vi "main.vi"() -> ()   [LabVIEW 2014]
uses:
  <vilib>/Utility/cursorutil.llb/Set Cursor (Icon Pict).vi
  <vilib>/vision/NI_Vision_Development_Module.lvlib
panel:
  out "DXF图":T1(plugin-control)
  out "填充效果":T1(plugin-control)
  out "文本":string
  in  "DXF文件路径":path
  out "数组":bool[][](array[boolean])
  out "未处理图像":T1(plugin-control)
  # "Usage: (1) The program written in LabVIEW 2014, you need to install NI Vision (2) First open the dxf path\n           (3) after the operation shows dxf graphics, in the \"DXF\" interface, the mouse click where you need to fill can\n                be automatically filled\nNote: DXF only supports \"segment\", \"circle\", \"arc\", rectangle or polygon needs to be decomposed into DXF, DXF is \n          saved, ellipse and elliptical arc are not supported"
  # "DXF图像填充器"
  # "使用方法：（1）本程序在LabVIEW 2014中编写，需要安装NI Vision（2）先打开dxf路径\n               （3）运行之后显示出dxf图形，在“DXF图”界面鼠标点击需要填充的地方即可实现自动填充\n注意：dxf图中仅支持“线段”、“圆”、“圆弧”，矩形或多边形需要分解爆炸成线段后保存DXF，不支持椭圆及椭圆弧"
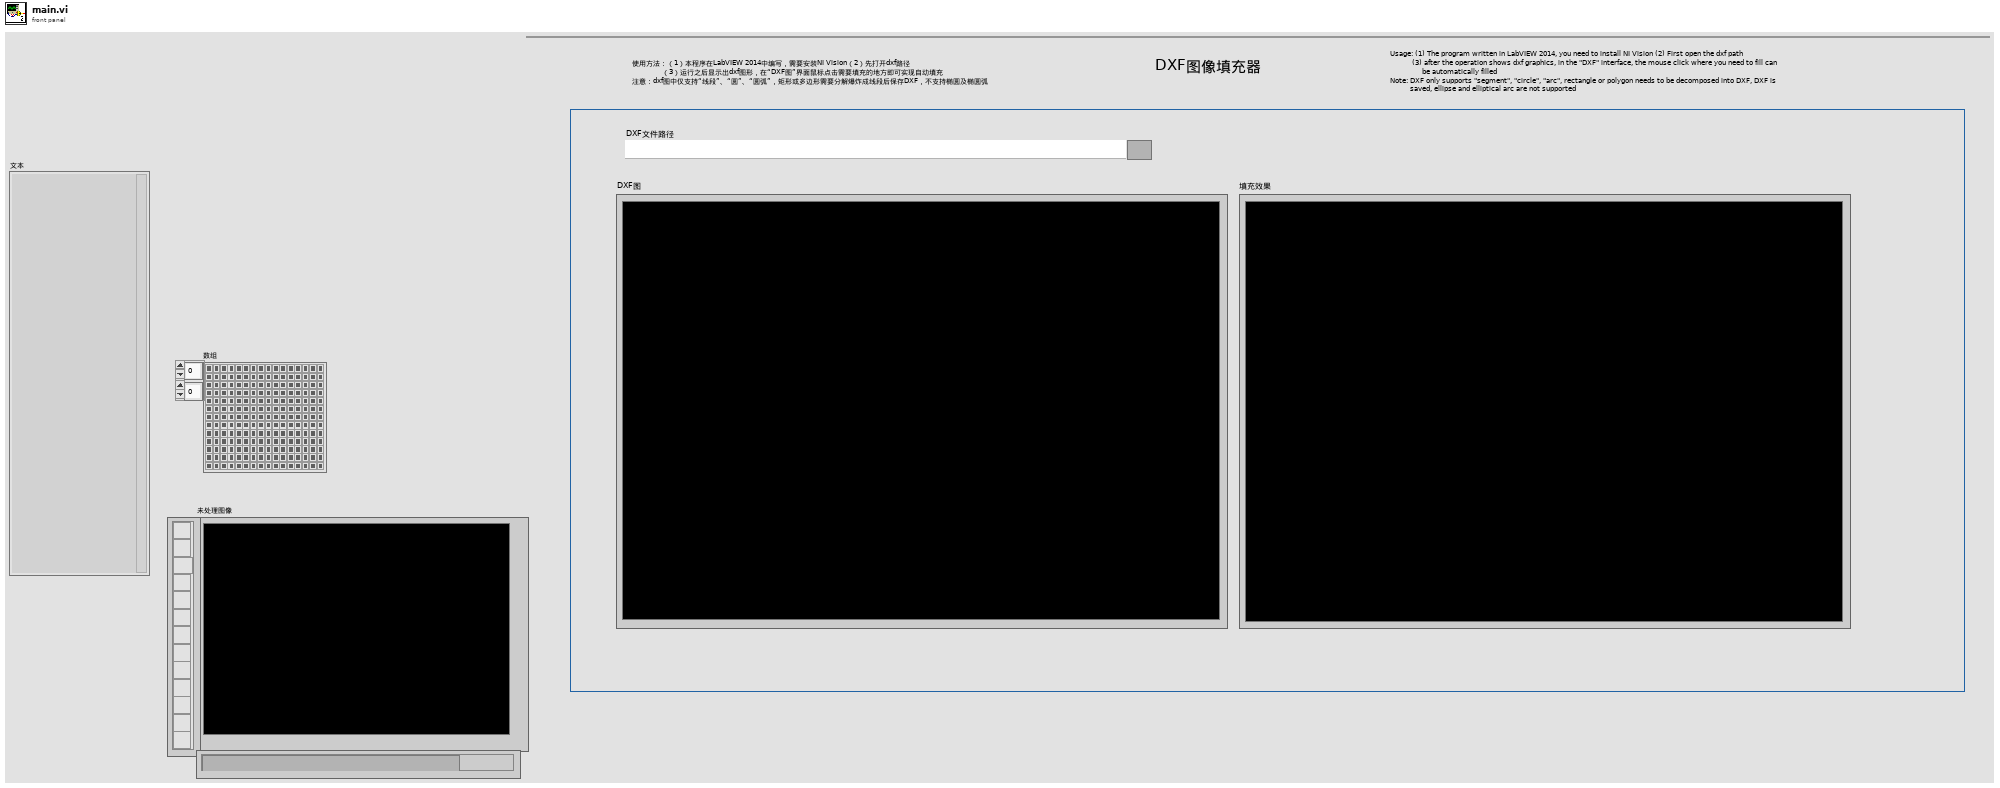
[diagram p1: front panel]
types:
  T1 = typedef "IMAQ Image.ctl" = refnum<image>
  T2 = enum32{"Solid", "Dash", "Dot", "DashDot", "DashDotDot"}
  T3 = cluster{"Width":u16, "Style":enum32{"Solid", "Dash", "Dot", "DashDot", "DashDotDot"}}
  T4 = cluster{"x":dbl, "y":dbl, "r":dbl, "start":dbl, "end":dbl}[]
  T5 = cluster{"线粗":u8, "Style":enum32{"Solid", "Dash", "Dot", "DashDot", "DashDotDot"}}
  T6 = cluster{"x":dbl, "y":dbl, "r":dbl, "start":dbl, "end":dbl}
  T7 = typedef "imagedata.ctl" = cluster{"image type":i32, "image depth":i32, "image":u8[], "mask":u8[], "colors":u32[], "Rectangle":cluster{"left":i16, "top":i16, "right":i16, "bottom":i16}}
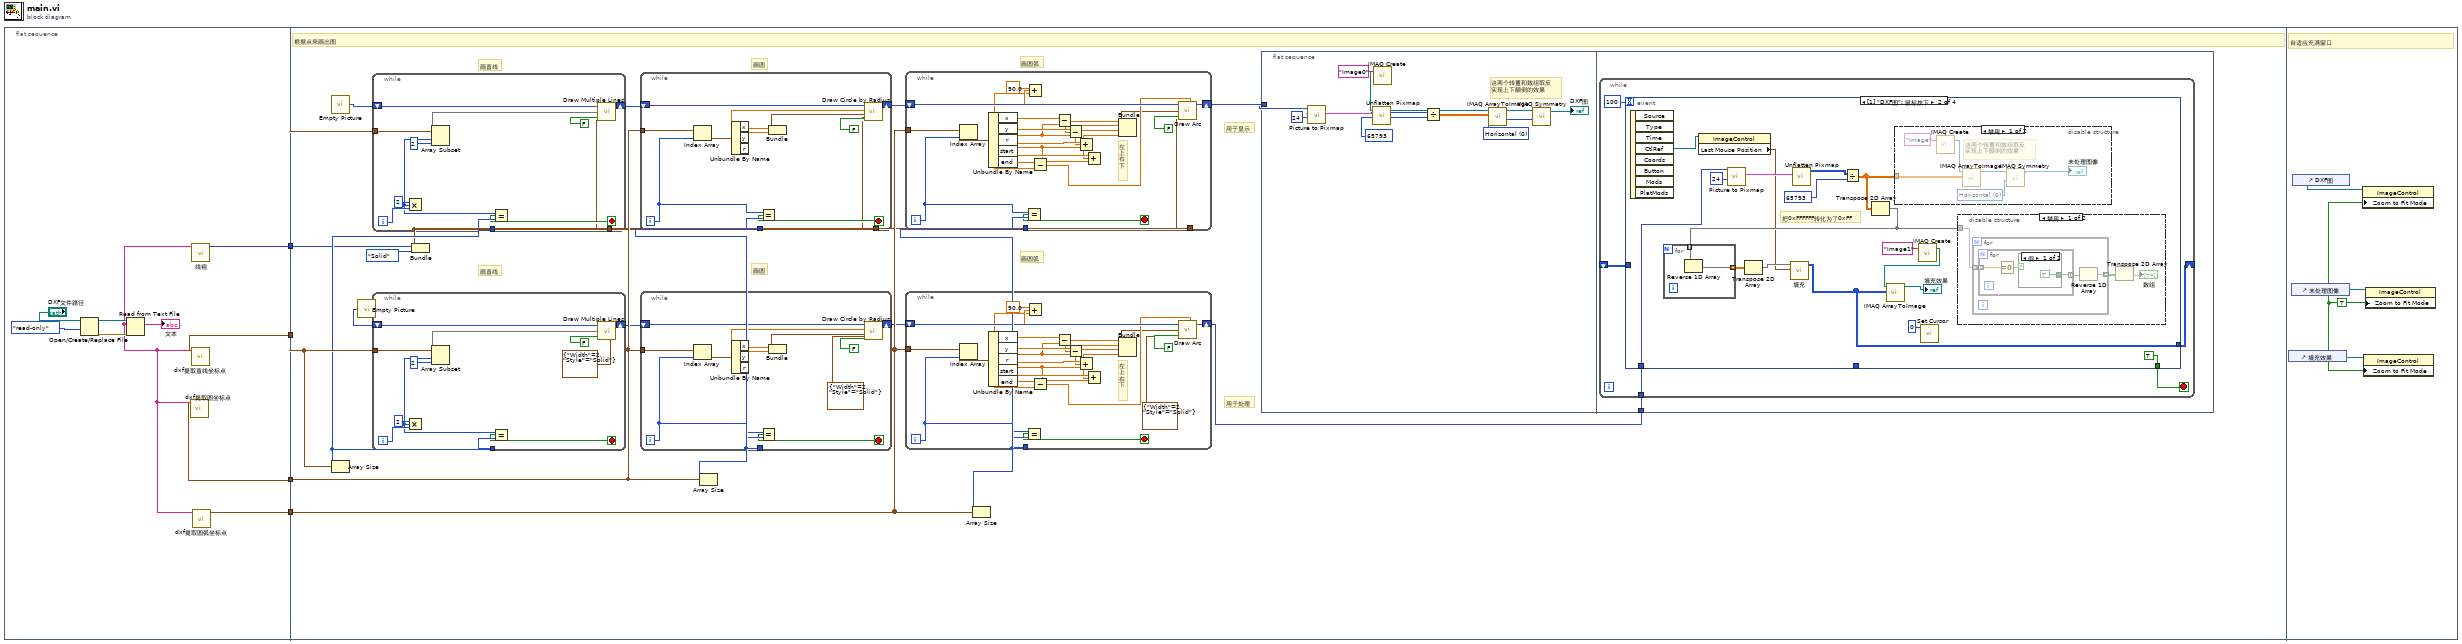
[diagram p0: block diagram]
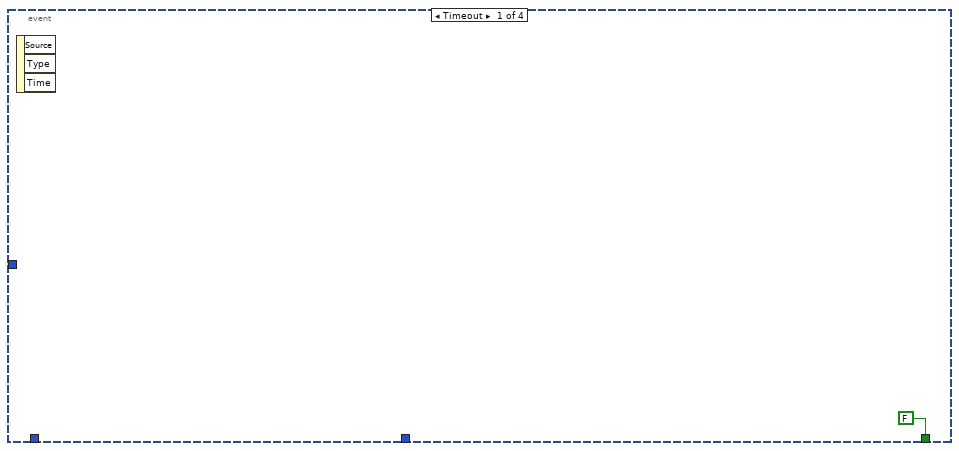
[diagram p2: hidden frame]
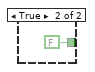
[diagram p4: hidden frame]
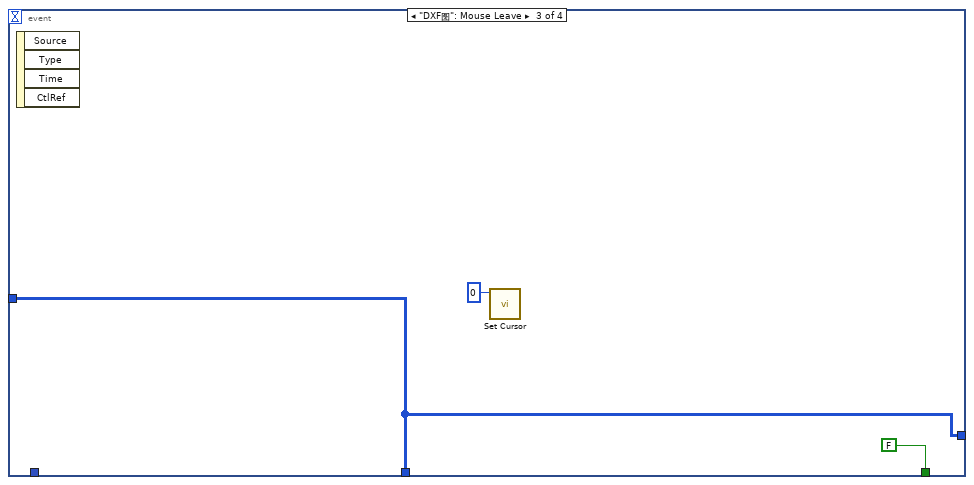
[diagram p6: hidden frame]
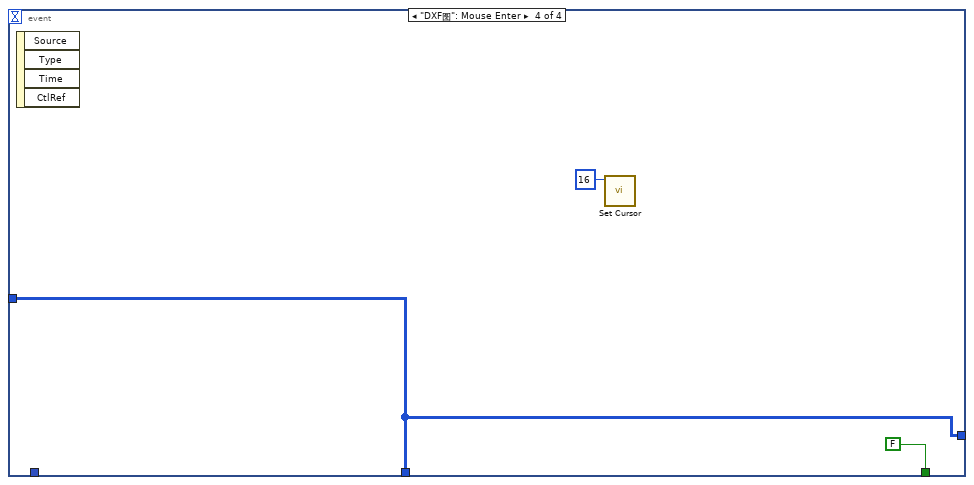
[diagram p7: hidden frame]
diagram:
  n1 = flat-sequence {
    tunnel: [w9] -> w4
    tunnel: [w8] -> w3
    tunnel: [w7] -> w2
    tunnel: [w5] -> w1
    tunnel: w4 -> [w25]
    tunnel: w3 -> [w26]
    tunnel: w2 -> [w27]
    tunnel: w1 -> [w18]
    frame #0 {
      n2 = Open/Create/Replace File(file path (use dialog)="DXF文件路径", access (0:read/write)=enum16{"read/write", "read-only", "write-only"}."read-only" ("权限(0:read/write)")) -> (refnum out=w11:refnum<file>, error out=w10:errorcluster)  [unwired: 4 in, 1 out]
      n3 = Read from Text File(file (use dialog)=w11, error in=w10) -> (text=w6:string)  [unwired: 2 in, 3 out]
      "文本" <- w6
      n4 = call "dxf提取圆坐标点.vi"("字符串"=w6) -> ("输出数组"=w8:cluster{"x":dbl, "y":dbl, "r":dbl}[])  [unwired: 10 in]
      n5 = call "dxf提取直线坐标点.vi"("字符串"=w6) -> ("数组"=w9:cluster{i32, i32}[])  [unwired: 10 in]
      n6 = call "线粗.vi"("字符串"=w6) -> ("线粗"=w5:u8)  [unwired: 10 in]
      n7 = call "dxf提取圆弧坐标点.vi"("字符串"=w6) -> ("输出数组"=w7:T4)  [unwired: 10 in]
    }
    frame #1 {
      # "画圆"
      # "画直线"
      # "用于显示"
      # "用于处理"
      # "画圆弧"
      # "画圆"
      # "画直线"
      # "画圆弧"
      # "根据点来画出图"
      n8 = call "Empty Picture"() -> ("empty picture"=w28:picture)
      n9 = Array Size(array=w25) -> (size(s)=w24:i32)
      n10 = call "Empty Picture"() -> ("empty picture"=w17:picture)
      n11 = while {
        shift-right: [w76] -> w16
        shift-left: w17 -> [w71]
        tunnel: w25 -> [w75]
        tunnel: w24 -> [w69]
        i -> [w74]
        stop <- w68 stop-if-true
        n12 = Multiply(x=2, y=w74) -> (x*y=w70:i32)
        n13 = Array Subset(array=w75, index=w70, length=2 ("长度")) -> (w66:cluster{i32, i32}[])
        n14 = Equal?(x=w70, y=w69) -> (x = y?=w68:bool)
        n15 = call <vilib>:"Draw Multiple Lines.vi"("picture"=w71, "line endpoints"=w66, "fill?(F)"=FALSE, "pen"=T3 {"Width"=2, "Style"=enum."Solid"}) -> ("new picture"=w76:picture)  [unwired: 5 in]
      }
      n16 = Bundle("线粗"=w18, "Style"=T2."Solid") -> (w20:T5)  [unwired: 1 in]
      n17 = while {
        shift-right: [w184] -> w29
        shift-left: w28 -> [w179]
        tunnel: w25 -> [w183]
        tunnel: w24 -> [w177]
        tunnel: w20 -> [w173]
        i -> [w182]
        stop <- w176 stop-if-true
        n18 = Multiply(x=2, y=w182) -> (x*y=w178:i32)
        n19 = Array Subset(array=w183, index=w178, length=2 ("长度")) -> (w174:cluster{i32, i32}[])
        n20 = Equal?(x=w178, y=w177) -> (x = y?=w176:bool)
        n21 = call <vilib>:"Draw Multiple Lines.vi"("picture"=w179, "line endpoints"=w174, "fill?(F)"=FALSE, "pen"=w173) -> ("new picture"=w184:picture)  [unwired: 5 in]
      }
      n22 = Array Size(array=w26) -> (size(s)=w23:i32)
      n23 = while {
        shift-right: [w170] -> w30
        shift-left: w29 -> [w169]
        tunnel: w26 -> [w168]
        tunnel: w23 -> [w172]
        tunnel: w20 -> [w160]
        i -> [w167]
        stop <- w171 stop-if-true
        n24 = Index Array(array=w168, index=w167) -> (element=w166:cluster{"x":dbl, "y":dbl, "r":dbl})
        n25 = Unbundle By Name(w166) -> ("x"=w163:dbl, "y"=w162:dbl, "r"=w165:dbl)
        n26 = Equal?(x=w167, y=w172) -> (x = y?=w171:bool)
        n27 = Bundle("x"=w163, "y"=w162) -> (w161:cluster{"x":dbl, "y":dbl})  [unwired: 1 in]
        n28 = call <vilib>:"Draw Circle by Radius.vi"("pen"=w160, "fill?(F)"=FALSE, "pixel center"=w161, "radius"=w165, "picture"=w169) -> ("new picture"=w170:picture)  [unwired: 6 in]
      }
      n29 = while {
        shift-right: [w63] -> w15
        shift-left: w16 -> [w62]
        tunnel: w26 -> [w61]
        tunnel: w23 -> [w65]
        i -> [w60]
        stop <- w64 stop-if-true
        n30 = Index Array(array=w61, index=w60) -> (element=w59:cluster{"x":dbl, "y":dbl, "r":dbl})
        n31 = Unbundle By Name(w59) -> ("x"=w56:dbl, "y"=w55:dbl, "r"=w58:dbl)
        n32 = Equal?(x=w60, y=w65) -> (x = y?=w64:bool)
        n33 = Bundle("x"=w56, "y"=w55) -> (w54:cluster{"x":dbl, "y":dbl})  [unwired: 1 in]
        n34 = call <vilib>:"Draw Circle by Radius.vi"("pen"=T3 {"Width"=2, "Style"=enum."Solid"}, "fill?(F)"=FALSE, "pixel center"=w54, "radius"=w58, "picture"=w62) -> ("new picture"=w63:picture)  [unwired: 6 in]
      }
      n35 = Array Size(array=w27) -> (size(s)=w22:i32)
      n36 = while {
        shift-right: [w157] -> w19
        shift-left: w30 -> [w156]
        tunnel: w27 -> [w155]
        tunnel: w22 -> [w159]
        tunnel: w20 -> [w138]
        i -> [w154]
        stop <- w158 stop-if-true
        # "左\n上\n右\n下"
        n37 = Index Array(array=w155, index=w154) -> (element=w153:T6)
        n38 = Unbundle By Name(w153) -> ("x"=w149:dbl, "y"=w148:dbl, "r"=w147:dbl, "start"=w140:dbl, "end"=w151:dbl)
        n39 = Equal?(x=w154, y=w159) -> (x = y?=w158:bool)
        n40 = Add(x=90.0, y=w140) -> (x+y=w141:dbl)
        n41 = Subtract(x=w151, y=w140) -> (x-y=w150:dbl)
        n42 = Subtract(x=w149, y=w147) -> (x-y=w146:dbl)
        n43 = Subtract(x=w148, y=w147) -> (x-y=w145:dbl)
        n44 = Add(x=w149, y=w147) -> (x+y=w144:dbl)
        n45 = Add(x=w148, y=w147) -> (x+y=w143:dbl)
        n46 = Bundle(w146, w145, w144, w143) -> (w142:cluster{dbl, dbl, dbl, dbl})  [unwired: 1 in]
        n47 = call <vilib>:"Draw Arc.vi"("picture"=w156, "start angle[degrees]"=w141, "rect"=w142, "fill?(F)"=FALSE, "arc size[degrees]"=w150, "pen"=w138) -> ("new picture"=w157:picture)  [unwired: 3 in]
      }
      n48 = while {
        shift-right: [w50] -> w14
        shift-left: w15 -> [w49]
        tunnel: w27 -> [w48]
        tunnel: w22 -> [w52]
        i -> [w47]
        stop <- w51 stop-if-true
        # "左\n上\n右\n下"
        n49 = Index Array(array=w48, index=w47) -> (element=w46:T6)
        n50 = Unbundle By Name(w46) -> ("x"=w41:dbl, "y"=w40:dbl, "r"=w39:dbl, "start"=w32:dbl, "end"=w43:dbl)
        n51 = Equal?(x=w47, y=w52) -> (x = y?=w51:bool)
        n52 = Add(x=90.0, y=w32) -> (x+y=w33:dbl)
        n53 = Subtract(x=w43, y=w32) -> (x-y=w42:dbl)
        n54 = Subtract(x=w41, y=w39) -> (x-y=w38:dbl)
        n55 = Subtract(x=w40, y=w39) -> (x-y=w37:dbl)
        n56 = Add(x=w41, y=w39) -> (x+y=w36:dbl)
        n57 = Add(x=w40, y=w39) -> (x+y=w35:dbl)
        n58 = Bundle(w38, w37, w36, w35) -> (w34:cluster{dbl, dbl, dbl, dbl})  [unwired: 1 in]
        n59 = call <vilib>:"Draw Arc.vi"("picture"=w49, "start angle[degrees]"=w33, "rect"=w34, "fill?(F)"=FALSE, "arc size[degrees]"=w42, "pen"=T3 {"Width"=2, "Style"=enum."Solid"}) -> ("new picture"=w50:picture)  [unwired: 3 in]
      }
      n60 = flat-sequence {
        tunnel: w19 -> [w80]
        tunnel: w14 -> [w89]
        frame #0 {
          w87 = u32 0 items=["Horizontal", "Vertical", "Central", "1st Diagonal", "2nd Diagonal"] ("Type of Symmetry")
          # "这两个转置和数组取反\n实现上下颠倒的效果"
          n61 = call <vilib>:"Picture to Pixmap.vi"("depth"=24, "picture"=w80) -> ("image data"=w81:T7)  [unwired: 8 in, 1 out]
          n62 = call <vilib>:"Unflatten Pixmap.vi"("image data"=w81) -> ("24-bit pixmap"=w83:u32[][])  [unwired: 4 in, 6 out]
          n63 = call "IMAQ Create"("Image Name"="Image0") -> ("New Image"=w84:T1)  [unwired: 4 in, 1 out]
          n64 = Divide(x=w83, y=65793) -> (x/y=w88:dbl[][])
          n65 = call "IMAQ ArrayToImage"("Image Pixels (U8)"=w88, "Image"=w84) -> ("Image Out"=w86:T1)  [unwired: 8 in, 1 out]
          n66 = call "IMAQ Symmetry"("Type of Symmetry"=w87, "Image Src"=w86) -> ("Image Dst Out"=→"DXF图":T1)  [unwired: 3 in, 1 out]
        }
        frame #1 {
          n67 = while {
            tunnel: w89 -> [w92]
            shift-right: [w91] -> _
            shift-left: _ -> [w90]
            stop <- w94 stop-if-true
            n68 = event shown="[1] \"DXF图\": 鼠标按下" {
              selector: _ -> [_ _ _ _]
              dyn-events: _ -> [_ _ _ _]
              timeout: 100 -> [_ _ _ _]
              tunnel: [FALSE TRUE FALSE FALSE] -> w94
              tunnel: w92 -> [_ w100 _ _]
              tunnel: [_ w96 w132 w135] -> w91
              tunnel: [_ _ w132 w135] -> _
              tunnel: w90 -> [_ _ w132 w135]
              event Timeout {
                n69 = event-data() -> ()  [unwired: 1 in, 3 out]
              }
              event "DXF图": Mouse Down {
                # "把0xFFFFFF转化为了0xFF"
                n70 = event-data() -> ("CtlRef"=w99:refnum<vi>)  [unwired: 1 in, 7 out]
                n71 = property class="ImageControl"(reference=w99) -> ("Last Mouse Position"=w98:cluster{"X":i32, "Y":i32})  [unwired: 1 in, 2 out]
                n72 = call <vilib>:"Picture to Pixmap.vi"("depth"=24, "picture"=w100) -> ("image data"=w103:T7)  [unwired: 8 in, 1 out]
                n73 = call <vilib>:"Unflatten Pixmap.vi"("image data"=w103) -> ("24-bit pixmap"=w104:u32[][])  [unwired: 4 in, 6 out]
                n74 = Divide(x=w104, y=65793) -> (x/y=w102:dbl[][])
                n75 = Transpose 2D Array(2D array=w102) -> (transposed array=w111:dbl[][])
                n76 = for {
                  tunnel: w111 -> [w131] mode=indexing
                  tunnel: [w130] -> w106 mode=indexing
                  n77 = Reverse 1D Array(array=w131) -> (reversed array=w130:dbl[])
                }
                n78 = Transpose 2D Array(2D array=w106) -> (transposed array=w112:dbl[][])
                n79 = call "填充.vi"("初始种子"=w98, "输入数组"=w112) -> ("输出数组"=w96:u8[][])  [unwired: 9 in]
                n80 = disable-structure shown="禁用" {
                  disable-tunnel: w102 -> [w113 _]
                  frame Disabled {
                    w116 = u32 0 items=["Horizontal", "Vertical", "Central", "1st Diagonal", "2nd Diagonal"] ("Type of Symmetry")
                    # "这两个转置和数组取反\n实现上下颠倒的效果"
                    n81 = call "IMAQ Create"("Image Name"="Image") -> ("New Image"=w114:T1)  [unwired: 4 in, 1 out]
                    n82 = call "IMAQ ArrayToImage"("Image Pixels (U8)"=w113, "Image"=w114) -> ("Image Out"=w117:T1)  [unwired: 8 in, 1 out]
                    n83 = call "IMAQ Symmetry"("Type of Symmetry"=w116, "Image Src"=w117) -> ("Image Dst Out"=→"未处理图像":T1)  [unwired: 3 in, 1 out]
                  }
                  frame Enabled {
                  }
                }
                n84 = call "IMAQ Create"("Image Name"="Image1") -> ("New Image"=w108:T1)  [unwired: 4 in, 1 out]
                n85 = call "IMAQ ArrayToImage"("Image Pixels (U8)"=w96, "Image"=w108) -> ("Image Out"=→"填充效果":T1)  [unwired: 8 in, 1 out]
                n86 = call-poly <vilib>:"Set Cursor.vi"("icon"=u16 0) -> ()  [unwired: 9 in, 2 out]
                n87 = disable-structure shown="禁用" {
                  disable-tunnel: w111 -> [w121 _]
                  frame Disabled {
                    n88 = for {
                      tunnel: [w123] -> w120 mode=indexing
                      tunnel: w121 -> [w122] mode=indexing
                      n89 = for {
                        tunnel: [w127] -> w124 mode=indexing
                        tunnel: w122 -> [w125] mode=indexing
                        n90 = Equal To 0?(x=w125) -> (x = 0?=w126:bool)
                        n91 = case shown="假" w126 {
                          tunnel: [TRUE FALSE] -> w127
                          frame False {
                          }
                          frame True {
                          }
                        }
                      }
                      n92 = Reverse 1D Array(array=w124) -> (reversed array=w123:bool[])
                    }
                    n93 = Transpose 2D Array(2D array=w120) -> (transposed array=→"数组":bool[][])
                  }
                  frame Enabled {
                  }
                }
              }
              event "DXF图": Mouse Leave {
                n94 = event-data() -> ()  [unwired: 1 in, 4 out]
                n95 = call-poly <vilib>:"Set Cursor.vi"("icon"=u16 0) -> ()  [unwired: 9 in, 2 out]
              }
              event "DXF图": Mouse Enter {
                n96 = event-data() -> ()  [unwired: 1 in, 4 out]
                n97 = call-poly <vilib>:"Set Cursor.vi"("icon"=u16 16) -> ()  [unwired: 9 in, 2 out]
              }
            }
          }
        }
      }
    }
    frame #2 {
      w185 = TRUE ("Zoom to Fit Mode")
      # "自适应充满窗口"
      n98 = control-ref of="填充效果"() -> (w186:refnum<vi>)
      n99 = control-ref of="未处理图像"() -> (w188:refnum<vi>)
      n100 = control-ref of="DXF图"() -> (w187:refnum<vi>)
      n101 = property class="ImageControl"(reference=w187, "Zoom to Fit Mode"=w185) -> ()  [unwired: 1 in, 2 out]
      n102 = property class="ImageControl"(reference=w186, "Zoom to Fit Mode"=w185) -> ()  [unwired: 1 in, 2 out]
      n103 = property class="ImageControl"(reference=w188, "Zoom to Fit Mode"=w185) -> ()  [unwired: 1 in, 2 out]
    }
  }
